vi "launcher.vi"   [LabVIEW 2023]
uses:
  <vilib>/ActorFramework/Actor/Actor.lvclass
  InterferometryUI/InterferometryUI.lvclass
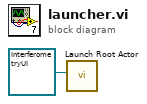
[diagram p0: block diagram]
diagram:
  n1 = call <vilib>:"Launch Root Actor.vi"("Actor"=refnum<class "InterferometryUI.lvclass"> refnum ("InterferometryUI.lvlib:InterferometryUI.lvclass")) -> ()  [unwired: 9 in, 2 out]
